vi "Retrieve Hierarchy.vi"(4 "Error in":errorcluster, 7 "Top-level VI path":path) -> (0 "Error out":errorcluster, 2 "# of VIs in hierarchy":i32, 3 "VIs in Hierarchy":path[](array[path]))   [LabVIEW 2010]
doc: "This Example Program searches for all the subVIs in the hierarchy of a given VI and returns an array of their paths. \nEach subVI is returned once in the list, regardless of how may times it appears in the hierarchy. \n\nClick on the browse button and select the VI whose hierarchy you want to find. Then run the program. You will receive the number of subVIs in the VI's hierarchy and an array that contains their paths."
uses:
  <vilib>/Utility/file.llb/Write To Spreadsheet File (string).vi
panel:
  out "Top-level VI refnum":refnum<vi>
  # "This Example Program searches for all the subVIs in the hierarchy of a given VI and returns an array \nof their paths. Each subVI is returned once in the list, regardless of how may times it appears in the \nhierarchy.  \n\nClick on the browse button and select the VI whose hierarchy you want to find. Then run the program.\nYou will receive the number of subVIs in the VI's hierarchy and an array that contains their paths."
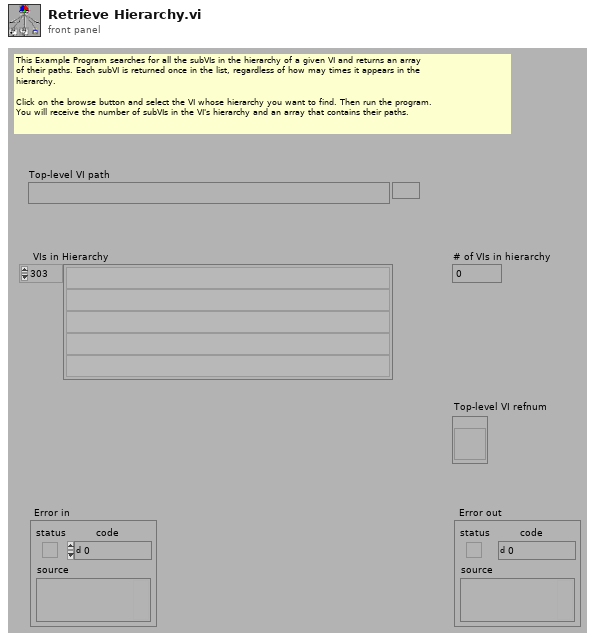
[diagram p1: front panel]
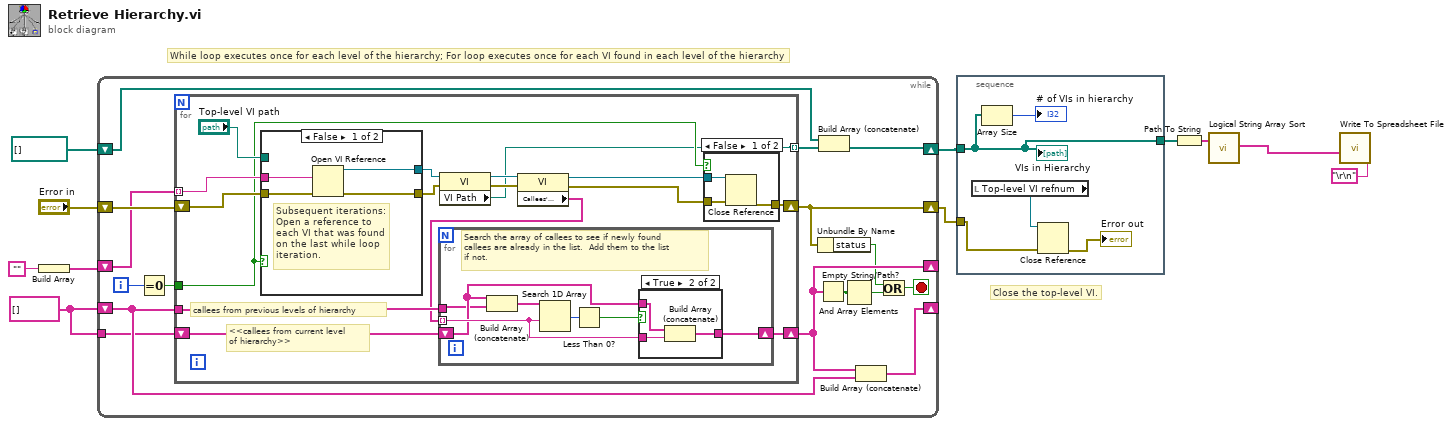
[diagram p0: block diagram]
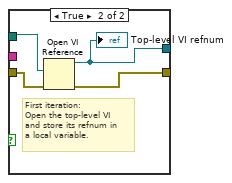
[diagram p4: hidden frame]
diagram:
  w7 = string[] []
  # "Close the top-level VI."
  # "While loop executes once for each level of the hierarchy; For loop executes once for each VI found in each level of the hierarchy"
  n1 = Build Array("") -> (w9:string[])
  n2 = while {
    tunnel: w7 -> [w16]
    shift-left: w7 -> [w17]
    shift-right: [w19] -> _
    shift-left: w9 -> [w22]
    shift-right: [w18] -> _
    shift-left: path[] [] -> [w26]
    shift-right: [w25] -> w8
    shift-left: "Error in" -> [w27]
    shift-right: [w21] -> w5
    i -> [w23]
    stop <- w12 stop-if-true
    n3 = Equal To 0?(x=w23) -> (x = 0?=w20:bool)
    n4 = for {
      shift-right: [w43] -> w21
      shift-left: w27 -> [w40]
      tunnel: w22 -> [w41] mode=indexing
      shift-right: [w38] -> w18
      shift-left: w16 -> [w39]
      tunnel: [w29] -> w15 mode=indexing
      tunnel: w20 -> [w36]
      tunnel: w17 -> [w35]
      # "callees from previous levels of hierarchy"
      # "<<callees from current level \nof hierarchy>>"
      n5 = case shown="False" w36 {
        tunnel: "Top-level VI path" -> [_ w65]
        tunnel: [w60 w63] -> w37
        tunnel: w41 -> [w59 _]
        tunnel: w40 -> [w62 w64]
        tunnel: [w61 w66] -> w28
        frame False {
          # "Subsequent iterations:\nOpen a reference to \neach VI that was found\non the last while loop \niteration."
          n6 = Open VI Reference(vi path=w59, error in (no error)=w62) -> (vi reference=w60:refnum<vi>, error out=w61:errorcluster)  [unwired: 4 in]
        }
        frame True {
          # "First iteration:  \nOpen the top-level VI\nand store its refnum in\na local variable."
          n7 = Open VI Reference(vi path=w65, error in (no error)=w64) -> (vi reference=w63:refnum<vi>, error out=w66:errorcluster)  [unwired: 4 in]
          "Top-level VI refnum" <- w63
        }
      }
      n8 = property class="VI"(reference=w37, error in=w28) -> (reference out=w34:refnum<vi>, error out=w33:errorcluster, "VI Path"=w29:path)
      n9 = property class="VI"(reference=w34, error in=w33) -> (reference out=w32:refnum<vi>, error out=w31:errorcluster, "Callees' Names"=w30:string[])
      n10 = for {
        tunnel: w30 -> [w52] mode=indexing
        shift-right: [w51] -> w38
        shift-left: w39 -> [w49]
        tunnel: w35 -> [w48]
        # "Search the array of callees to see if newly found \ncallees are already in the list.  Add them to the list \nif not."
        n11 = Build Array (concatenate)(w49, w48) -> (w50:string[])
        n12 = Search 1D Array(1D array=w50, element=w52) -> (index of element=w54:i32)  [unwired: 1 in]
        n13 = Less Than 0?(x=w54) -> (x < 0?=w53:bool)
        n14 = case shown="True" w53 {
          tunnel: w49 -> [w55 w58]
          tunnel: w52 -> [_ w57]
          tunnel: [w55 w56] -> w51
          frame False {
          }
          frame True {
            n15 = Build Array (concatenate)(w58, w57) -> (w56:string[])
          }
        }
      }
      n16 = case shown="False" w36 {
        tunnel: [w46 w47] -> w43
        tunnel: w31 -> [w45 w47]
        tunnel: w32 -> [w44 _]
        frame False {
          n17 = Close Reference(reference=w44, error in (no error)=w45) -> (error out=w46:errorcluster)
        }
        frame True {
        }
      }
    }
    n18 = Unbundle By Name(w21) -> ("status"=w13:bool)
    n19 = Empty String/Path?(string/path=w18) -> (empty?=w24:bool[])
    n20 = Build Array (concatenate)(w26, w15) -> (w25:path[])
    n21 = And Array Elements(Boolean array=w24) -> (logical AND=w14:bool)
    n22 = Build Array (concatenate)(w18, w17) -> (w19:string[])
    n23 = Or(x=w13, y=w14) -> (x .or. y?=w12:bool)
  }
  n24 = stacked-sequence {
    tunnel: w8 -> [w67]
    tunnel: w5 -> [w69]
    tunnel: [w67] -> w4
    frame #0 {
      n25 = local read "Top-level VI refnum"() -> (w70:refnum<vi>)
      n26 = Array Size(array=w67) -> (size(s)=→"# of VIs in hierarchy":i32)
      n27 = Close Reference(reference=w70, error in (no error)=w69) -> (error out=→"Error out":errorcluster)
      "VIs in Hierarchy" <- w67
    }
  }
  n28 = Path To String(path=w4) -> (string=w2:string[])
  n29 = call "Logical String Array Sort.vi"("Unsorted List"=w2) -> ("Sorted List"=w1:string[])  [unwired: 18 in]
  n30 = call-poly <vilib>:"Write To Spreadsheet File.vi"("delimiter (\\t)"="\r\n", "1D data"=w1) -> ()  [unwired: 6 in, 1 out]
